vi "onListenForNewConnection.vi"(8 "error in (no error)":errorcluster, 9 "timeout (ms)":i32=1, 11 "Listener":refnum<class "Connection.LocalQueue.lvclass">) -> (0 "error out":errorcluster, 1 "New connection":bool, 2 "timed out":bool, 3 "New Connection":refnum<class "Connection.lvclass">)   [LabVIEW 2013, in "Connection.Queue_GOSPL.lvlib" / "Connection.LocalQueue.lvclass"]
uses:
  Connection.LocalQueue.lvclass
  Connection/Connection.lvclass
  Connection.LocalQueue.lvclass/Connection.LocalQueue.ctl
  <vilib>/LabVIEW Open Source Project/Unicity/RandomStringGenerator/RandomStringGenerator.lvclass
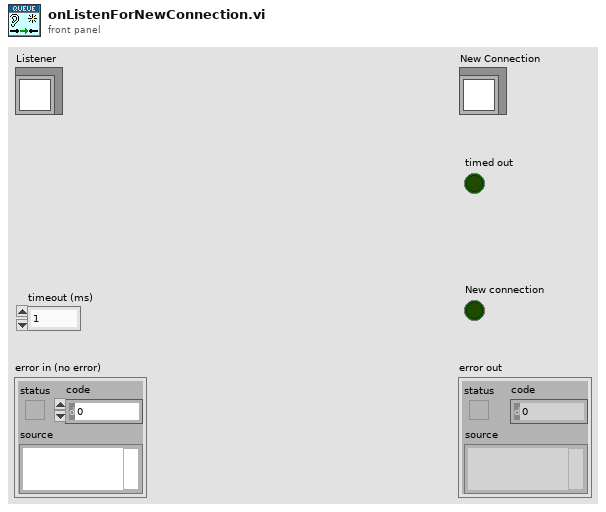
[diagram p1: front panel]
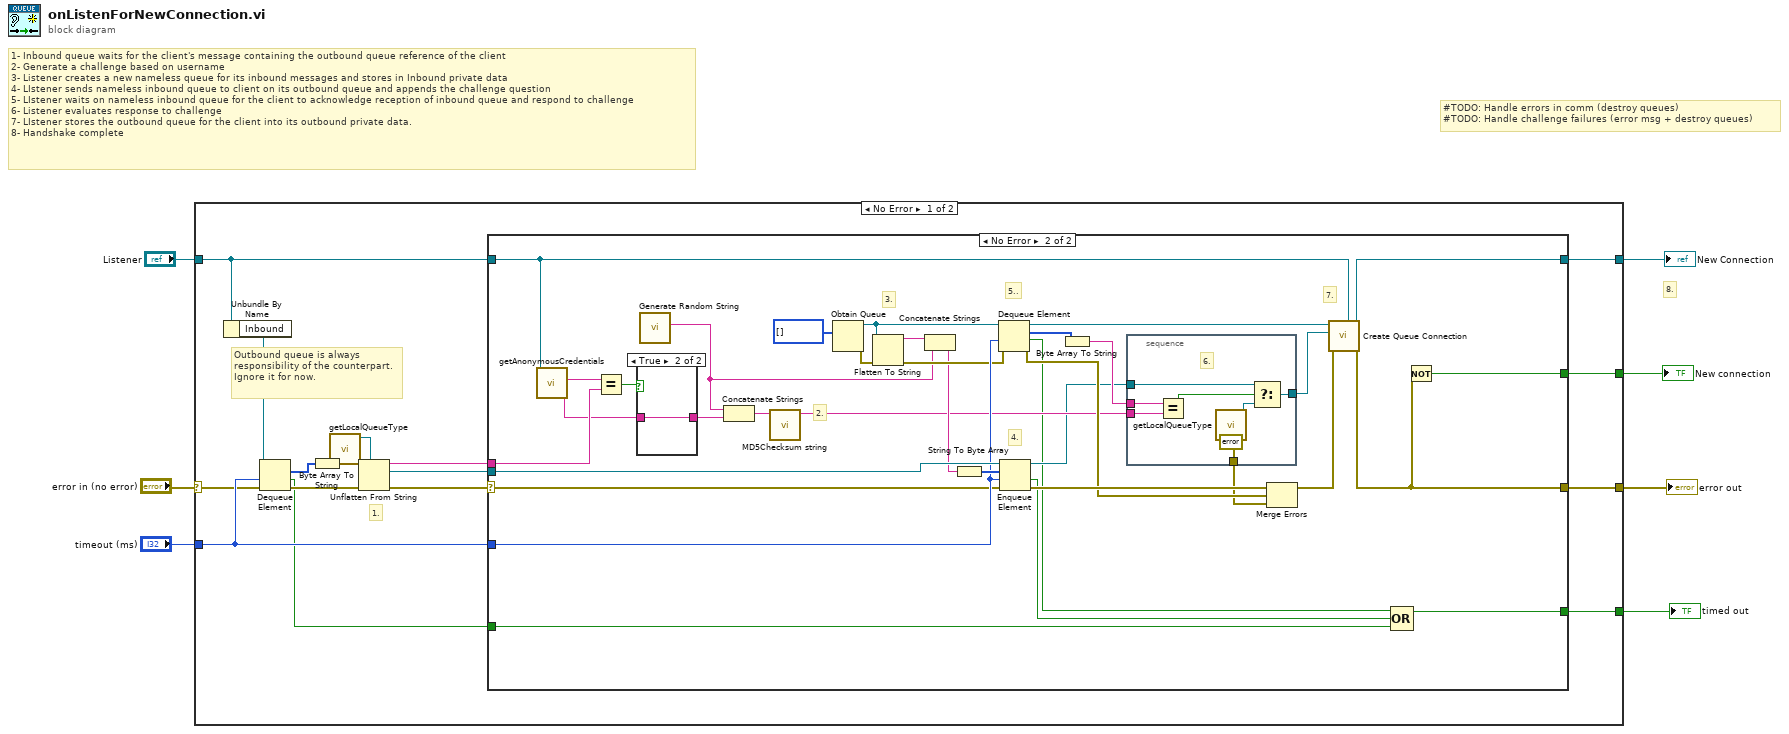
[diagram p0: block diagram]
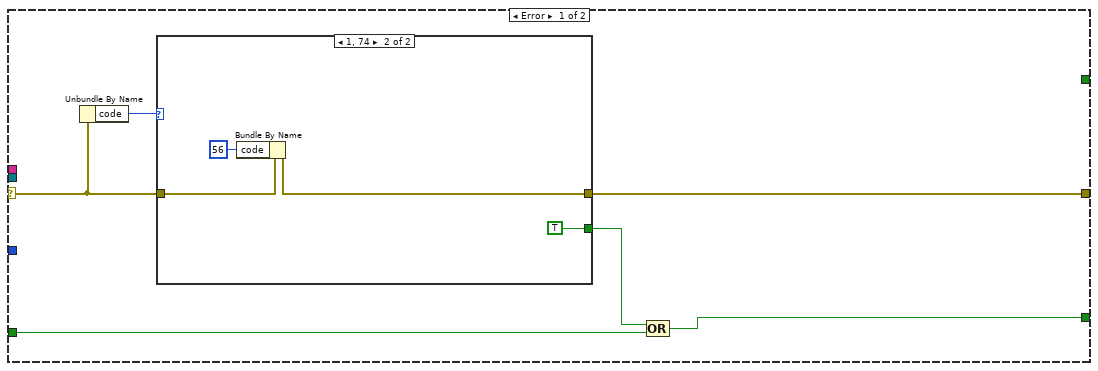
[diagram p2: hidden frame]
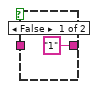
[diagram p4: hidden frame]
diagram:
  # "#TODO: Handle errors in comm (destroy queues)\n#TODO: Handle challenge failures (error msg + destroy queues)"
  # "8."
  # "1- Inbound queue waits for the client's message containing the outbound queue reference of the client\n2- Generate a challenge based on username\n3- Listener creates a new nameless queue for its inbound messages and stores in Inbound private data\n4- LIstener sends nameless inbound queue to client on its outbound queue and appends the challenge question\n5- LIstener waits on nameless inbound queue for the client to acknowledge reception of inbound queue and respond to challenge\n6- Listener evaluates response to challenge\n7- LIstener stores the outbound queue for the client into its outbound private data.\n8- Handshake complete"
  n1 = case shown="No Error" "error in (no error)" {
    selector: "error in (no error)" -> [w8 w79]
    tunnel: [w23 _] -> w7
    tunnel: "timeout (ms)" -> [w17 _]
    tunnel: [w16 w79] -> w5
    tunnel: [w14 _] -> w4
    tunnel: [w12 _] -> w3
    tunnel: "Listener" -> [w10 _]
    frame No Error {
      # "Outbound queue is always responsibility of the counterpart. Ignore it for now."
      # "1."
      n2 = Unbundle By Name(w10) -> ("Inbound"=w21:refnum<queue>)
      n3 = Dequeue Element(queue=w21, timeout in ms (-1)=w17, error in (no error)=w8) -> (element=w22:u8[], timed out?=w11:bool, error out=w19:errorcluster)  [unwired: 1 out]
      n4 = Byte Array To String(unsigned byte array=w22) -> (string=w20:string)
      n5 = call "getLocalQueueType.vi"() -> ("Queue Type"=w15:refnum<queue>)  [unwired: 11 in]
      n6 = Unflatten From String(type=w15, binary string=w20, error in (no error)=w19) -> (rest of the binary string=w13:string, value=w18:refnum<queue>, error out=w9:errorcluster)  [unwired: 2 in]
      n7 = case shown="No Error" w9 {
        selector: w9 -> [w28 w35]
        tunnel: [_ w69] -> w23
        tunnel: w18 -> [_ w65]
        tunnel: w17 -> [_ w63]
        tunnel: [w27 w61] -> w16
        tunnel: [_ w52] -> w14
        tunnel: w13 -> [_ w48]
        tunnel: [w25 w40] -> w12
        tunnel: w11 -> [w26 w37]
        tunnel: w10 -> [_ w36]
        frame Error {
          n8 = Unbundle By Name(w28) -> ("code"=w29:i32)
          n9 = case shown="1, 74" w29 {
            tunnel: w28 -> [w30 w34]
            tunnel: [w30 w32] -> w27
            tunnel: [_ TRUE] -> w24
            frame Default {
            }
            frame 1, 74 {
              n10 = Bundle By Name(cluster=w34, "code"=56) -> (w32:errorcluster)
            }
          }
          n11 = Compound Arithmetic op=OR(w24, w26) -> (w25:bool)
        }
        frame No Error {
          # "2."
          # "3."
          # "7."
          # "5.."
          # "4."
          n12 = call "getAnonymousCredentials.vi"("Connection.LocalQueue"=w36) -> ("Anonymous password"=w44:string, "Anonymous username"=w51:string)  [unwired: 9 in]
          n13 = Equal?(x=w51, y=w48) -> (x = y?=w46:bool)
          n14 = case shown="True" w46 {
            tunnel: ["1" ("Anonymous password") w71] -> w45
            tunnel: w44 -> [_ w71]
            frame False {
            }
            frame True {
            }
          }
          n15 = call <vilib>:"Generate Random String.vi"() -> ("Random String"=w47:string)  [unwired: 11 in]
          n16 = Concatenate Strings(w47, w45) -> (w50:string)
          n17 = call <vilib>:"MD5Checksum string.vi"("Message String"=w50) -> ("MD5 message-digest"=w49:string)  [unwired: 10 in]
          n18 = Obtain Queue(element data type=u8[] [] ("element")) -> (queue out=w60:refnum<queue>, error out=w59:errorcluster)  [unwired: 4 in, 1 out]
          n19 = Flatten To String(anything=w60, error in (no error)=w59) -> (data string=w56:string, error out=w58:errorcluster)  [unwired: 2 in, 1 out]
          n20 = Concatenate Strings(w56, w47) -> (w53:string)
          n21 = String To Byte Array(string=w53) -> (unsigned byte array=w68:u8[])
          n22 = Dequeue Element(queue=w60, timeout in ms (-1)=w63, error in (no error)=w58) -> (queue out=w64:refnum<queue>, element=w55:u8[], timed out?=w39:bool, error out=w57:errorcluster)
          n23 = Enqueue Element(queue=w65, element=w68, timeout in ms (-1)=w63, error in (no error)=w35) -> (queue out=w42:refnum<queue>, timed out?=w38:bool, error out=w67:errorcluster)
          n24 = Byte Array To String(unsigned byte array=w55) -> (string=w54:string)
          n25 = stacked-sequence {
            tunnel: w54 -> [w77]
            tunnel: w49 -> [w78]
            tunnel: [errorcluster {"status"=FALSE, "code"=0, "source"=""} ("error in")] -> w43
            tunnel: w42 -> [w75]
            tunnel: [w74] -> w41
            frame #0 {
              # "6."
              n26 = Equal?(x=w77, y=w78) -> (x = y?=w73:bool)
              n27 = call "getLocalQueueType.vi"() -> ("Queue Type"=w72:refnum<queue>)  [unwired: 11 in]
              n28 = Select(t=w75, s=w73, f=w72) -> (s? t:f=w74:refnum<queue>)
            }
          }
          n29 = Merge Errors(w67, w57, w43) -> (w62:errorcluster)
          n30 = call "Create Queue Connection.vi"("Connection.LocalQueue"=w36, "error in (no error)"=w62, "Outbound"=w41, "Inbound"=w64) -> ("error out"=w61:errorcluster, "Connection.LocalQueue"=w52:refnum<class "Connection.LocalQueue.lvclass">)  [unwired: 6 in]
          n31 = Compound Arithmetic op=OR(w39, w38, w37) -> (w40:bool)
          n32 = Not(x=w61) -> (.not. x?=w69:bool)
        }
      }
    }
    frame Error {
    }
  }
  "error out" <- w5
  "New Connection" <- w4
  "New connection" <- w7
  "timed out" <- w3
